vi "PQ Example COPY.vi"() -> ()   [LabVIEW 2016]
uses:
  Connection/PQ Connection.lvclass
panel:
  in  "table name":string="test11"
  in  "connection string":string
  out "x-y":dbl
  in  "delimiter (Tab)":string="\t"
  out "buffer":string
  in  "Strings":string[][](array[string])
  out "error out":errorcluster
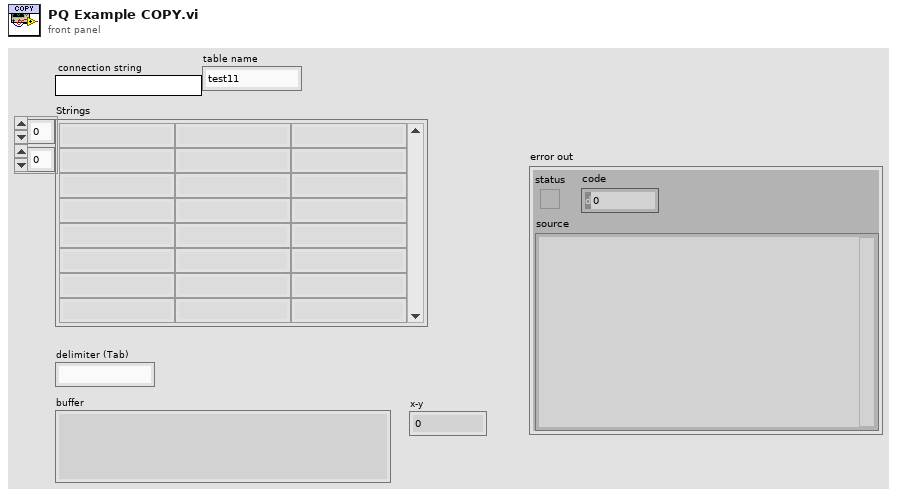
[diagram p1: front panel]
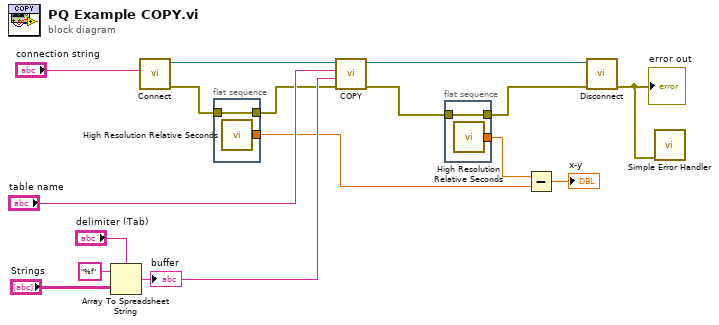
[diagram p0: block diagram]
diagram:
  n1 = Array To Spreadsheet String(delimiter (Tab)="delimiter (Tab)", array="Strings", 3:"%f" ("format string")) -> (spreadsheet string=w13:string)
  "buffer" <- w13
  n2 = call "Connect.vi"("Connection Strings"="connection string") -> ("error out"=w11:errorcluster, "PQ Connection out"=w8:refnum<class "PQ Connection.lvclass">)  [unwired: 9 in]
  n3 = flat-sequence {
    tunnel: w11 -> [w18]
    tunnel: [w18] -> w5
    tunnel: [w17] -> w3
    frame #0 {
      n4 = call <vilib>:"High Resolution Relative Seconds.vi"() -> ("relative seconds"=w17:dbl)
    }
  }
  n5 = call "COPY.vi"("error in (no error)"=w5, "buffer"=w13, "table name"="table name", "PQ Connection in"=w8) -> ("error out"=w9:errorcluster, "PQ Connection out"=w6:refnum<class "PQ Connection.lvclass">)  [unwired: 6 in]
  n6 = flat-sequence {
    tunnel: w9 -> [w20]
    tunnel: [w20] -> w10
    tunnel: [w19] -> w4
    frame #0 {
      n7 = call <vilib>:"High Resolution Relative Seconds.vi"() -> ("relative seconds"=w19:dbl)
    }
  }
  n8 = Subtract(x=w4, y=w3) -> (x-y=→"x-y":dbl)
  n9 = call-dynamic "Disconnect.vi"("error in (no error)"=w10, "PQ Connection in"=w6) -> ("error out"=w12:errorcluster)  [unwired: 9 in]
  "error out" <- w12
  n10 = call <vilib>:"Simple Error Handler.vi"("error in (no error)"=w12) -> ()  [unwired: 4 in, 5 out]
